vi "remove_waveforms.vi"(5 "Enable Analout Output":bool, 8 "error in (no error)":errorcluster, 9 "analog output DAQmx task":refnum<k21>) -> (0 "error out":errorcluster)   [LabVIEW 2013]
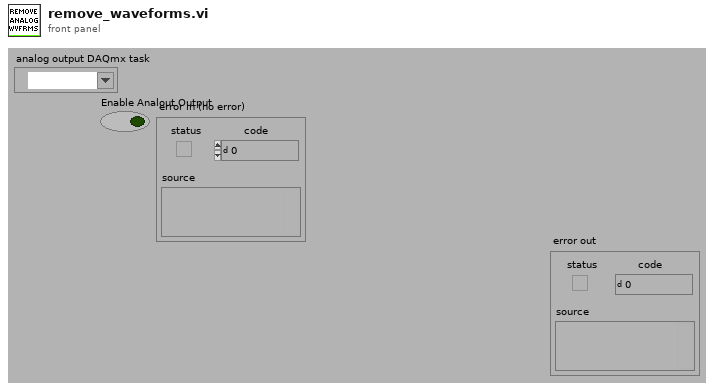
[diagram p1: front panel]
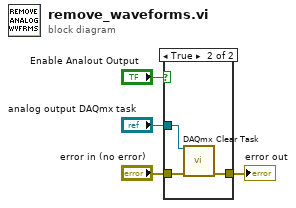
[diagram p0: block diagram]
diagram:
  n1 = case shown="True" "Enable Analout Output" {
    tunnel: "analog output DAQmx task" -> [_ w8]
    tunnel: [w5 w7] -> w2
    tunnel: "error in (no error)" -> [w5 w6]
    frame False {
    }
    frame True {
      n2 = call <vilib>:"DAQmx Clear Task.vi"("task in"=w8, "error in"=w6) -> ("error out"=w7:errorcluster)  [unwired: 13 out]
    }
  }
  "error out" <- w2
